vi "Multiscale Pyramids Cleaned Up.vi"() -> ()   [LabVIEW 2023]
uses:
  Images/_Images.ctl
  SubVIs/Multiscale Parameters Typedef.ctl
  SubVIs/Conv Flt Presets.ctl
  SubVIs/Unsharp Mask Params TypeDef.ctl
  SubVIs/ImagesPool Operations TypeDef.ctl
  SubVIs/Parameters Operations.ctl
  <vilib>/vision/NI_Vision_Development_Module.lvlib
panel:
  in  "Load":bool
  in  "Save":bool
  in  "MultiScale Parameters":T1={"Preprocessing"=enum."Convolution", "Convolution"=enum."Seifert 5x5", "Unsharp Mask Params"={"Amount"=6.0, "Radius"=33.0, "Threshold"=30.0}, "LUT Power"=[0.61538464, 0.43076923, 0.3846154, 0.43846154, 0.42307693, 0.5538462, 0.64615387, 0.61538464, 0.61538464, 0.6, 0.4, 0.4], "LUT Multiplier"=[157.53847, 185.1077, 192.98462, 248.12308, 196.92308, 248.12308, 252.06154, 114.215385, 248.12308, 110.276924, 102.4, 102.4], "Filters"=[enum."Seifert 7x7", enum."Seifert 5x5", enum."Highlight Details 3x3", enum."None", enum."None", enum."None", enum."None", enum."None", enum."None", enum."None", enum."None", enum."None"], "X Value PostProc"=1.2} {"X Value PostProc" scale=0.75..3.0; "LUT Multiplier" scale=0.0..512.0; "LUT Power" scale=0.0..2.0}
  in  "stop":bool
  out "Time, ms":u32
  out "Histogram":T4(graph)
  out "Reconstructed\nImage":T5(plugin-control)
  out "Source Image":T5(plugin-control)
  in  "Image":T6=enum."Part1"
  # "Multiscale Contrast Enhancement using Pyramids"
  # "1024x1024"
  # "2048x2048"
  # "4096x4096"
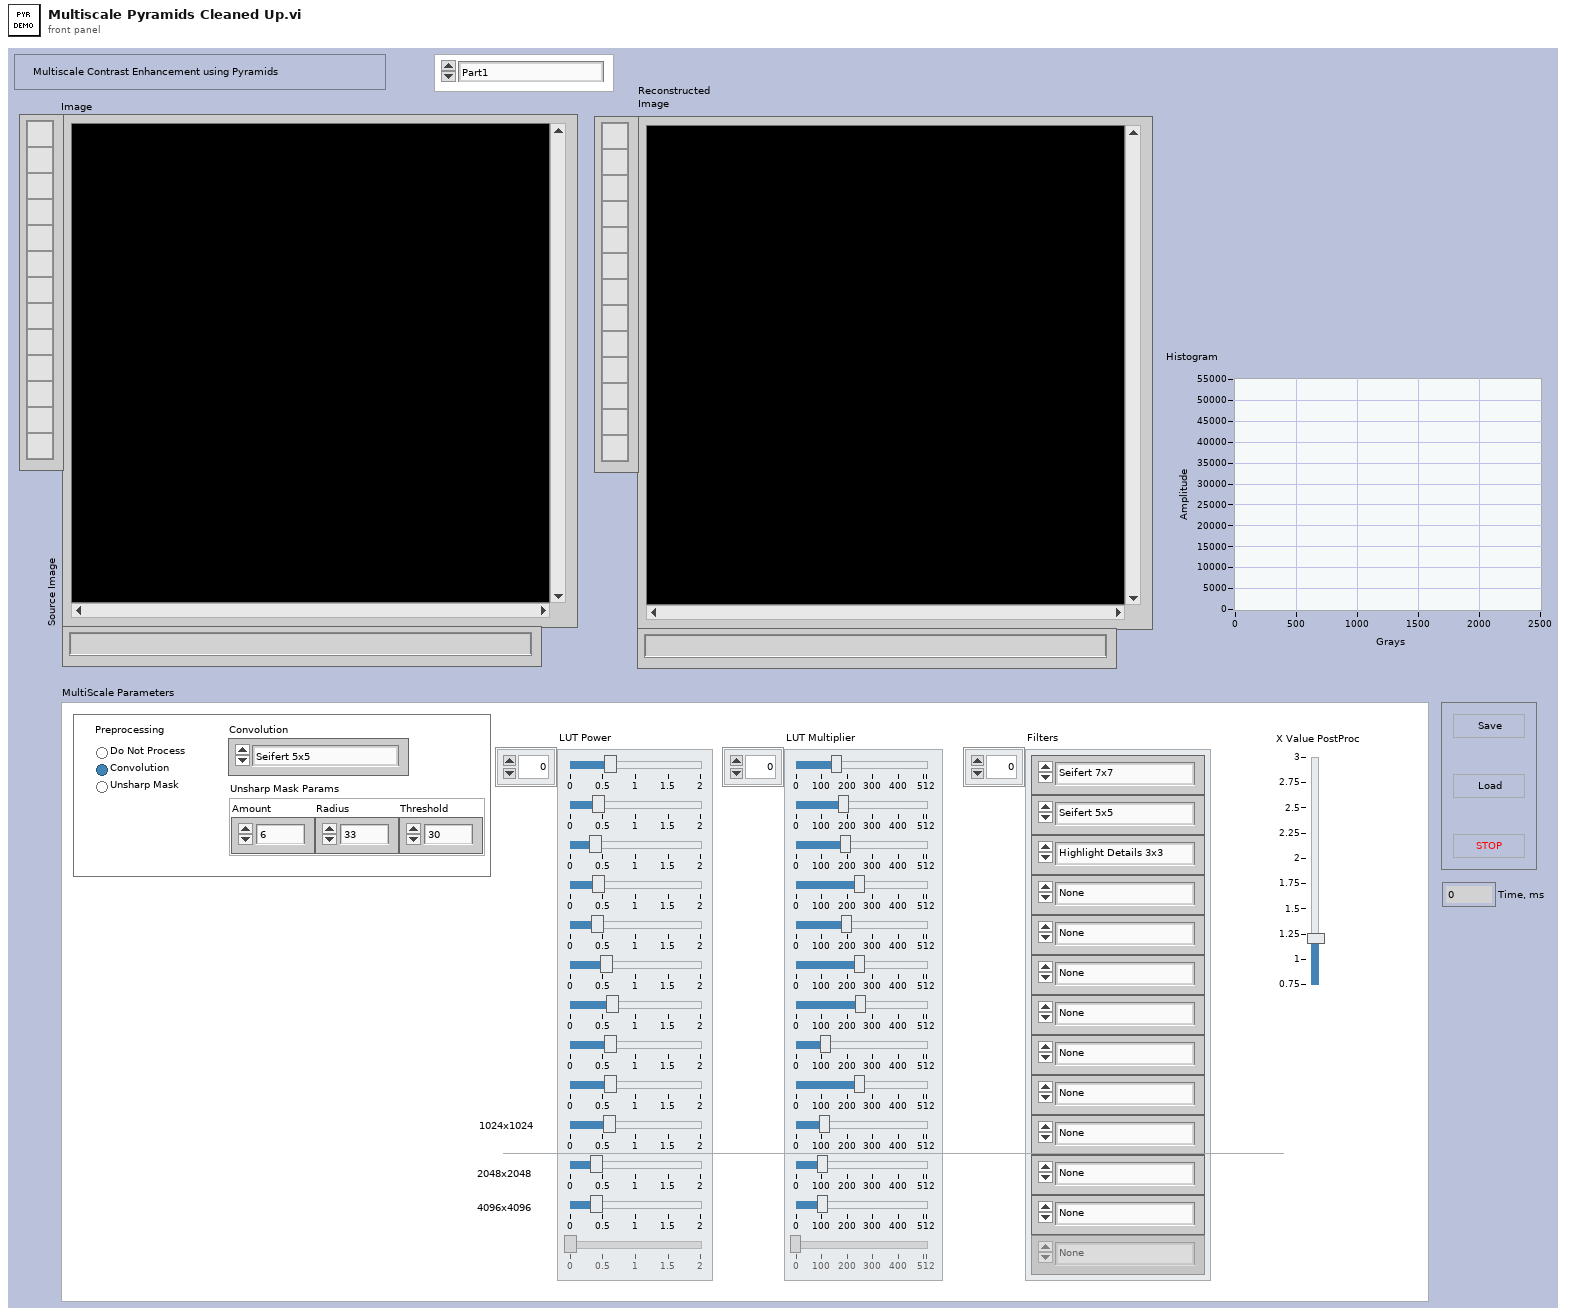
[diagram p1: front panel]
types:
  T1 = typedef "Multiscale Parameters Typedef.ctl" = cluster{"Preprocessing":enum32{"Do Not Process", "Convolution", "Unsharp Mask"}, "Convolution":T2, "Unsharp Mask Params":T3, "LUT Power":sgl[], "LUT Multiplier":sgl[], "Filters":T2[], "X Value PostProc":sgl}
  T2 = typedef "Conv Flt Presets.ctl" = enum16{"None", "Seifert 5x5", "Seifert 7x7", "High Pass 5x5 ", "High Pass 7x7", "Highlight Details 3x3", "Highlight Details 5x5", "Highlight Detail 7x7"}
  T3 = typedef "Unsharp Mask Params TypeDef.ctl" = cluster{"Amount":sgl, "Radius":sgl, "Threshold":sgl}
  T4 = cluster{"Starting Value":sgl, "Incremental Value":sgl, "Histogram":u32[]}
  T5 = typedef "IMAQ Image.ctl" = refnum<image>
  T6 = typedef "_Images.ctl" = enum16{"Ostern2023", "Balls2", "Battery1", "Battery2", "Connector1", "Subwoofer1", "Subwoofer2", "Subwoofer3", "Subwoofer4", "Hase1", "Lamp1", "Lamp2", "Mouse1", "PhotoLens1", "Po1", "PowerSupply1", "Router", "--- Step Wedges ---", "Stepwedge1", "Stepwedge2", "Stepwedge3", "--- PART 01 ---", "Part1", "Part2", "Part3", "Part4", "Part5", "Part6", "Part7", "Part8"}
  T7 = typedef "ImagesPool Operations TypeDef.ctl" = enum16{"Init", "Get Image", "Dispose"}
  T8 = typedef "Image Type" = u32
  T9 = typedef "Parameters Operations.ctl" = enum16{"Init", "Get", "Apply", "Save to File", "Load from File"}
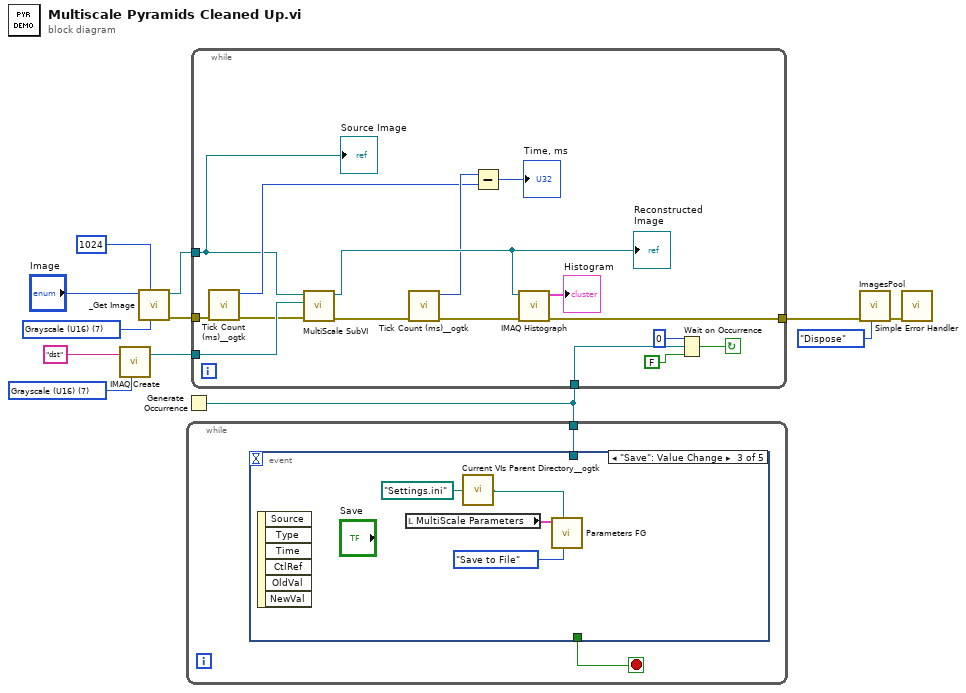
[diagram p0: block diagram]
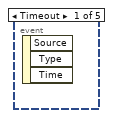
[diagram p2: hidden frame]
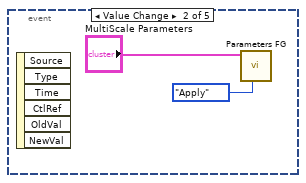
[diagram p3: hidden frame]
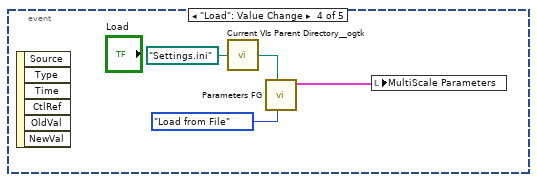
[diagram p4: hidden frame]
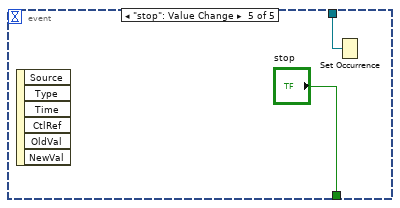
[diagram p5: hidden frame]
diagram:
  w9 = T8 7 items=["Grayscale (U8)", "Grayscale (I16)", "Grayscale (SGL)", "Complex (CSG)", "RGB (U32)", "HSL (U32)", "RGB (U64)", "Grayscale (U16)"] ("Image Type (U16)")
  w11 = T8 7 items=["Grayscale (U8)", "Grayscale (I16)", "Grayscale (SGL)", "Complex (CSG)", "RGB (U32)", "HSL (U32)", "RGB (U64)", "Grayscale (U16)"] ("Image Type")
  n1 = call "IMAQ Create"("Image Name"="dst", "Image Type"=w11) -> ("New Image"=w4:T5)  [unwired: 3 in, 1 out]
  n2 = call "_Get Image.vi"("Image Type (U16)"=w9, "XY Resolution"=1024, "Image"="Image") -> ("error out"=w7:errorcluster, "Image Out"=w6:T5)  [unwired: 5 in, 2 out]
  n3 = Generate Occurrence() -> (w5:refnum<k4>)
  n4 = while {
    tunnel: w5 -> [w13]
    stop <- w14 stop-if-true
    n5 = event shown="[2] \"Save\": Value Change" {
      selector: _ -> [_ _ _ _ _]
      dyn-events: _ -> [_ _ _ _ _]
      timeout: _ -> [_ _ _ _ _]
      tunnel: [_ _ _ _ "stop"] -> w14
      tunnel: w13 -> [_ _ _ _ w25]
      event Timeout {
        n6 = event-data() -> ()  [unwired: 1 in, 3 out]
      }
      event Value Change {
        n7 = event-data() -> ()  [unwired: 1 in, 6 out]
        n8 = call "Parameters FG.vi"("Params Operations (Get)"=Parameters_Operations."Apply" ("Params Operations"), "MultiScale Parameters In"="MultiScale Parameters") -> ()  [unwired: 8 in, 2 out]
      }
      event "Save": Value Change {
        n9 = event-data() -> ()  [unwired: 1 in, 6 out]
        n10 = local read "MultiScale Parameters"() -> (w19:T1)
        n11 = call <userlib>:"Current VIs Parent Directory__ogtk.vi"("Relative path (.)"=path "Settings.ini") -> ("Parent Directory (+ Relative)"=w17:path)  [unwired: 4 in]
        n12 = call "Parameters FG.vi"("Params Operations (Get)"=Parameters_Operations."Save to File", "configuration file path"=w17, "MultiScale Parameters In"=w19) -> ()  [unwired: 7 in, 2 out]
      }
      event "Load": Value Change {
        n13 = event-data() -> ()  [unwired: 1 in, 6 out]
        n14 = call <userlib>:"Current VIs Parent Directory__ogtk.vi"("Relative path (.)"=path "Settings.ini") -> ("Parent Directory (+ Relative)"=w21:path)  [unwired: 4 in]
        n15 = call "Parameters FG.vi"("Params Operations (Get)"=Parameters_Operations."Load from File", "configuration file path"=w21) -> ("MultiScale Parameters Out"=w23:T1)  [unwired: 8 in, 1 out]
        n16 = local write "MultiScale Parameters"(w23) -> ()
      }
      event "stop": Value Change {
        n17 = event-data() -> ()  [unwired: 1 in, 6 out]
        n18 = Set Occurrence(w25) -> ()
      }
    }
  }
  n19 = while {
    tunnel: w4 -> [w39]
    tunnel: w7 -> [w38]
    tunnel: w6 -> [w31]
    tunnel: [w35] -> w2
    tunnel: w5 -> [w34]
    stop <- w33 continue-if-true
    n20 = call <userlib>:"Tick Count (ms)__ogtk.vi"("error in (no error)"=w38) -> ("error out"=w28:errorcluster, "millisecond timer value"=w40:u32)  [unwired: 9 in]
    n21 = call "MultiScale SubVI.vi"("error in (no error)"=w28, "Image Dst"=w39, "Image Src"=w31) -> ("error out"=w30:errorcluster, "Image Dst Out"=w42:T5)  [unwired: 6 in, 1 out]
    "Reconstructed\nImage" <- w42
    n22 = call <userlib>:"Tick Count (ms)__ogtk.vi"("error in (no error)"=w30) -> ("error out"=w29:errorcluster, "millisecond timer value"=w41:u32)  [unwired: 9 in]
    n23 = Subtract(x=w41, y=w40) -> (x-y=→"Time, ms":u32)
    n24 = call "IMAQ Histograph"("error in (no error)"=w29, "Image"=w42) -> ("error out"=w35:errorcluster, "Histogram Graph"=→"Histogram":T4)  [unwired: 6 in, 2 out]
    n25 = Wait on Occurrence(1:FALSE ("ignore previous (T)"), 2:w34, 3:0 ("ms timeout (-1)")) -> (0:w33:bool)
    "Source Image" <- w31
  }
  n26 = call "ImagesPool.vi"("Op"=ImagesPool_Operations_TypeDef."Dispose", "error in (no error)"=w2) -> ("error out"=w1:errorcluster)  [unwired: 7 in, 2 out]
  n27 = call <vilib>:"Simple Error Handler.vi"("error in (no error)"=w1) -> ()  [unwired: 4 in, 5 out]
